vi "Xls export.vi"(6 "X Scale.Format String":string="%#.6g", 8 "error in (no error)":errorcluster, 11 "Wykres ref":refnum<vi>) -> (0 "error out":errorcluster)   [LabVIEW 2014]
doc: "Zapisuje dane z wykresu do pliku excella\nz poprawieniem rozdzielczoœci na osi oX\nwzglêdem ustalonej domyœlnie na wykresie"
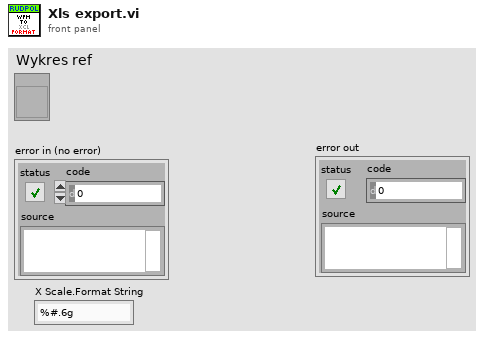
[diagram p1: front panel]
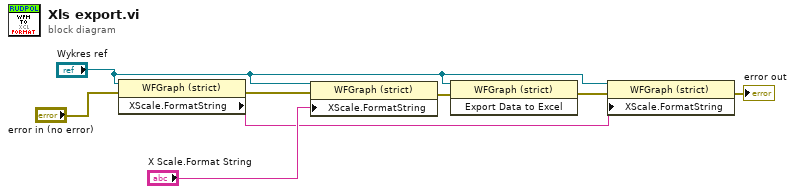
[diagram p0: block diagram]
diagram:
  n1 = property on="Property Node" class="WFGraph (strict)"(reference="Wykres ref", error in="error in (no error)") -> (error out=w7:errorcluster, "XScale.FormatString"=w4:string)  [unwired: 1 out]
  n2 = property on="Property Node" class="WFGraph (strict)"(reference="Wykres ref", error in=w7, "XScale.FormatString"="X Scale.Format String") -> (error out=w6:errorcluster)  [unwired: 1 out]
  n3 = invoke on="Invoke Node" class="WFGraph (strict)" method="Export Data to Excel"(reference="Wykres ref", error in=w6) -> (error out=w5:errorcluster)  [unwired: 1 in, 2 out]
  n4 = property on="Property Node" class="WFGraph (strict)"(reference="Wykres ref", error in=w5, "XScale.FormatString"=w4) -> (error out=→"error out":errorcluster)  [unwired: 1 out]
